vi "Iteration.vi"(7 "Total Iterations":i32=-1, 8 "error in (no error)":errorcluster, 9 "Current Iteration":i32=-1, 10 "Message":string, 11 "Progress Bar":refnum<data-value>) -> (0 "error out":errorcluster, 2 "Aborted":bool, 3 "Progress Bar":refnum<data-value>)   [LabVIEW 2016, in "Progress Bar.lvclass"]
doc: "This VI should be called every iteration of the loop. If the Progress Bar input is valid, it will use the configuration specified. If not, it will use the default config.\n\nIf current iteration is left unwired, it will keep track of the number of times it's been called to figure out where in the progress bar it is.\n\nCopyright: MGI\nAuthored by: Derek Trepanier"
uses:
  <userlib>/_MGI/User Interface/Progress Bar/Progress Bar.lvclass
  <userlib>/_MGI/User Interface/Progress Bar/Progress Bar.lvclass/Progress Bar.ctl
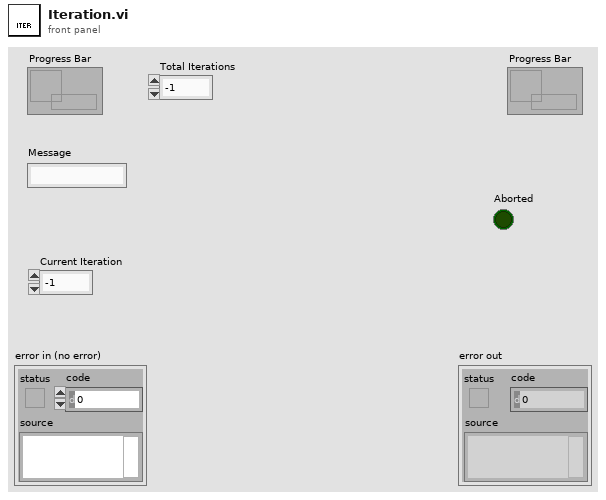
[diagram p1: front panel]
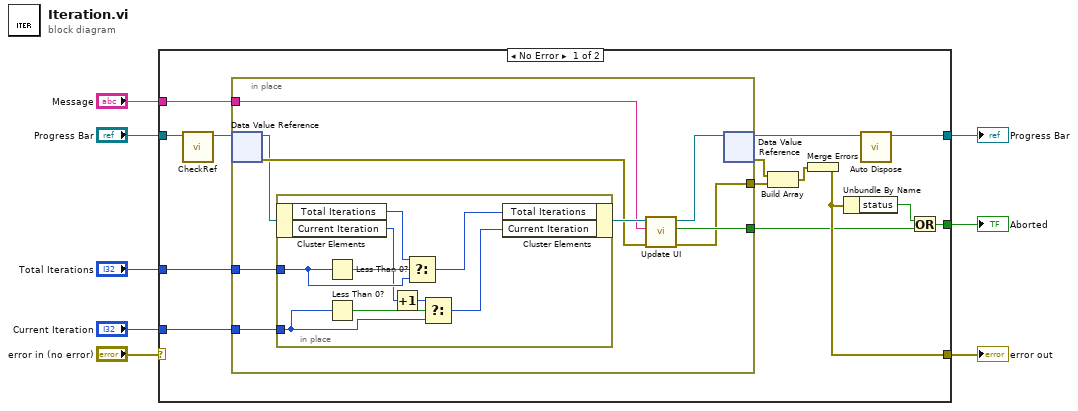
[diagram p0: block diagram]
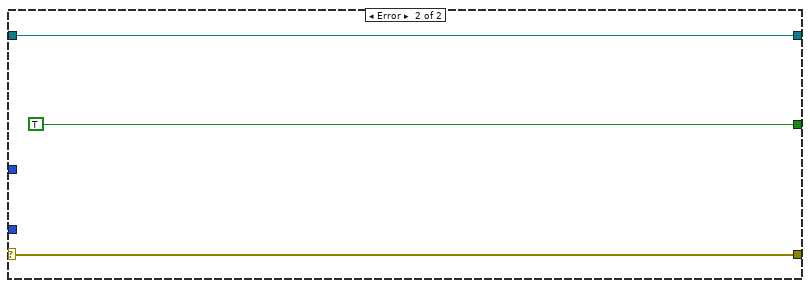
[diagram p2: hidden frame]
diagram:
  n1 = case shown="No Error" "error in (no error)" {
    selector: "error in (no error)" -> [_ w43]
    tunnel: [w18 w43] -> w7
    tunnel: [w12 w42] -> w6
    tunnel: "Progress Bar" -> [w15 w42]
    tunnel: "Total Iterations" -> [w22 _]
    tunnel: "Current Iteration" -> [w21 _]
    tunnel: [w17 TRUE] -> w2
    tunnel: "Message" -> [w11 _]
    frame No Error {
      n2 = call <userlib>:"CheckRef.vi"("Progress Bar"=w15) -> ("Progress Bar"=w14:refnum<data-value>)  [unwired: 9 in, 1 out]
      n3 = in-place {
        in-place-border: w22 -> [w31]
        in-place-border: w21 -> [w30]
        in-place-border: [w25] -> w19
        in-place-border: [w26] -> w16
        in-place-border: w11 -> [w24]
        n4 = in-place-dvr #1(w14) -> (w23:refnum<class "Progress Bar.lvclass">, w28:errorcluster)
        n5 = in-place {
          in-place-border: w31 -> [w38]
          in-place-border: w30 -> [w36]
          n6 = in-place-cluster #2(w23) -> ("Total Iterations"=w39:i32, "Current Iteration"=w35:i32)
          n7 = Less Than 0?(x=w38) -> (x < 0?=w40:bool)
          n8 = Less Than 0?(x=w36) -> (x < 0?=w37:bool)
          n9 = Increment(x=w35) -> (x+1=w32:i32)
          n10 = Select(t=w39, s=w40, f=w38) -> (s? t:f=w33:i32)
          n11 = Select(t=w32, s=w37, f=w36) -> (s? t:f=w34:i32)
          n12 = in-place-cluster #2("Total Iterations"=w33, "Current Iteration"=w34) -> (w29:refnum<class "Progress Bar.lvclass">)
        }
        n13 = call <userlib>:"Update UI.vi"("error in (no error)"=w28, "Message"=w24, "MGI_Progress Bar in"=w29) -> ("error out"=w25:errorcluster, "Aborted"=w26:bool, "MGI_Progress Bar out"=w27:refnum<class "Progress Bar.lvclass">)  [unwired: 6 in]
        n14 = in-place-dvr #1(w27) -> (w13:refnum<data-value>, w20:errorcluster)
      }
      n15 = Build Array(w20, w19) -> (w10:errorcluster[])
      n16 = Merge Errors(w10) -> (w18:errorcluster)
      n17 = Unbundle By Name(w18) -> ("status"=w9:bool)
      n18 = call <userlib>:"Auto Dispose.vi"("Progress Bar"=w13) -> ("Progress Bar"=w12:refnum<data-value>)  [unwired: 9 in, 1 out]
      n19 = Or(x=w9, y=w16) -> (x .or. y?=w17:bool)
    }
    frame Error {
    }
  }
  "error out" <- w7
  "Progress Bar" <- w6
  "Aborted" <- w2
